vi "Handle Events.vi"(8 "error in (no error)":errorcluster, 11 "ApplicationEventHandler":refnum<class "ApplicationEventHandler.lvclass">) -> ()   [LabVIEW 2015, in "ActorEvents.lvlib" / "ApplicationEventHandler.lvclass"]
uses:
  ApplicationEventHandler.lvclass
  IEventHandler/IEventHandler.lvclass/IEventHandler.ctl
  ApplicationEventHandler.lvclass/ApplicationEventHandler.ctl
  <vilib>/ActorFramework/Message Enqueuer/Message Enqueuer.lvclass/Message Enqueuer.ctl
  <vilib>/ActorFramework/Message Priority Queue/Priority Enqueue.vi
  IEventHandler/IEventHandler.lvclass
  <vilib>/ActorFramework/Message Enqueuer/Message Enqueuer.lvclass
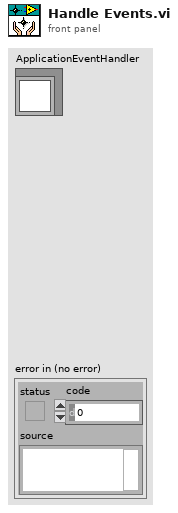
[diagram p1: front panel]
types:
  T1 = typedef "Actor Framework.lvlib/Message Enqueuer.lvclass/Message Priority.ctl" = enum16{"Low", "Normal", "High"}
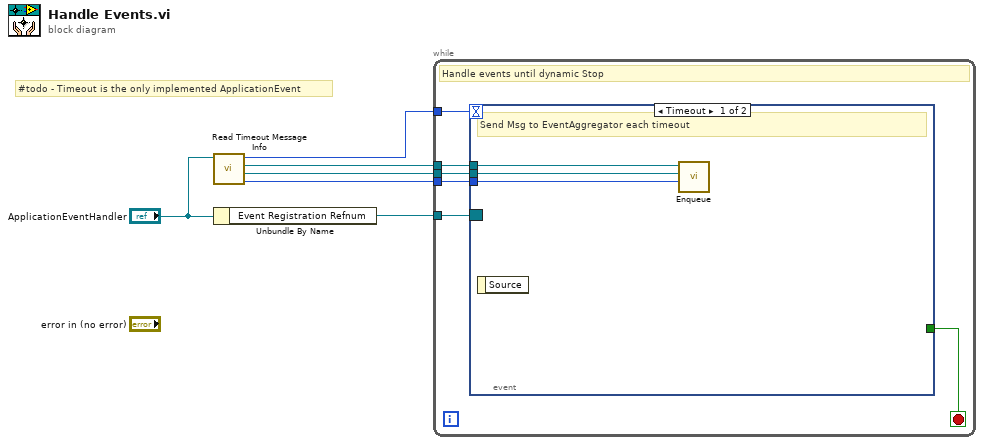
[diagram p0: block diagram]
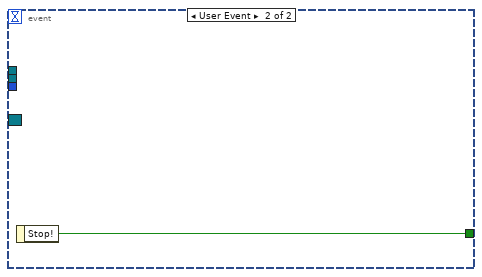
[diagram p2: hidden frame]
diagram:
  # "#todo - Timeout is the only implemented ApplicationEvent"
  n1 = call "Read Timeout Message Info.vi"("IEventHandler in"="ApplicationEventHandler") -> ("Timeout Message Priority"=w1:T1, "Timeout Message"=w2:refnum<class "Message.lvclass">, "EventAggregator Enqueuer"=w4:refnum<class "Message Enqueuer.lvclass">, "Timeout [ms]"=w3:i32)  [unwired: 7 in]
  n2 = Unbundle By Name("ApplicationEventHandler") -> ("Event Registration Refnum"=w6:refnum<event-registration>)
  n3 = while {
    tunnel: w6 -> [w12]
    tunnel: w2 -> [w11]
    tunnel: w3 -> [w10]
    tunnel: w4 -> [w8]
    tunnel: w1 -> [w7]
    stop <- w9 stop-if-true
    # "Handle events until dynamic Stop"
    n4 = event shown="[0] Timeout" {
      selector: w12 -> [_ _]
      dyn-events: _ -> [_ _]
      timeout: w10 -> [_ _]
      tunnel: w11 -> [w14 _]
      tunnel: [_ w16] -> w9
      tunnel: w8 -> [w15 _]
      tunnel: w7 -> [w13 _]
      event Timeout {
        # "Send Msg to EventAggregator each timeout"
        n5 = event-data() -> ()  [unwired: 1 in, 1 out]
        n6 = call <vilib>:"Enqueue.vi"("Message Priority (Normal)"=w13, "Message"=w14, "Message Enqueuer in"=w15) -> ()  [unwired: 7 in, 2 out]
      }
      event User Event {
        n7 = event-data() -> ("Stop!"=w16:bool)  [unwired: 1 in]
      }
    }
  }
